vi "8bit-arr-dec.vi"(11 "Array":bool[](array[boolean])) -> (3 "f":dbl)   [LabVIEW 2017]
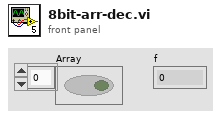
[diagram p1: front panel]
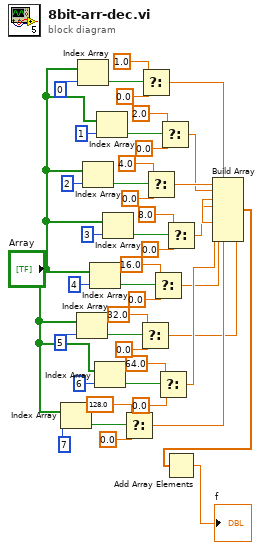
[diagram p0: block diagram]
diagram:
  n1 = Index Array(array="Array", index=7) -> (element=w32:bool)
  n2 = Index Array(array="Array", index=5) -> (element=w24:bool)
  n3 = Index Array(array="Array", index=0) -> (element=w4:bool)
  n4 = Index Array(array="Array", index=2) -> (element=w12:bool)
  n5 = Index Array(array="Array", index=4) -> (element=w20:bool)
  n6 = Index Array(array="Array", index=6) -> (element=w28:bool)
  n7 = Index Array(array="Array", index=1) -> (element=w8:bool)
  n8 = Index Array(array="Array", index=3) -> (element=w16:bool)
  n9 = Select(t=128.0, s=w32, f=0.0) -> (s? t:f=w41:dbl)
  n10 = Select(t=32.0, s=w24, f=0.0) -> (s? t:f=w39:dbl)
  n11 = Select(t=1.0, s=w4, f=0.0) -> (s? t:f=w34:dbl)
  n12 = Select(t=4.0, s=w12, f=0.0) -> (s? t:f=w36:dbl)
  n13 = Select(t=16.0, s=w20, f=0.0) -> (s? t:f=w38:dbl)
  n14 = Select(t=64.0, s=w28, f=0.0) -> (s? t:f=w40:dbl)
  n15 = Select(t=2.0, s=w8, f=0.0) -> (s? t:f=w35:dbl)
  n16 = Select(t=8.0, s=w16, f=0.0) -> (s? t:f=w37:dbl)
  n17 = Build Array(w34, w35, w36, w37, w38, w39, w40, w41) -> (w43:dbl[])
  n18 = Add Array Elements(numeric array=w43) -> (sum=→"f":dbl)
